vi "ScriptCreateEnumTypedef.vi"(9 "I/O names":string[](array[string]), 11 "Path to Saved File":path) -> ()   [LabVIEW 2014]
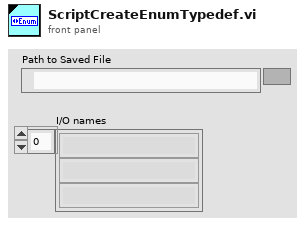
[diagram p1: front panel]
types:
  T1 = enum32{"not a control VI", "control", "typedef", "strict typedef"}
  T2 = enum32{"invalid VI type", "Standard VI", "Control VI", "Global VI", "Polymorphic VI", "Configuration VI", "SubSystem", "Facade VI", "Method VI", "Statechart Diagram VI"}
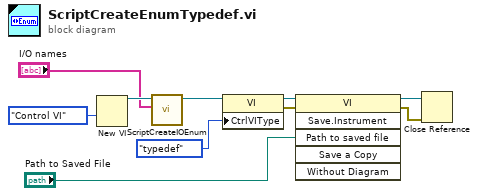
[diagram p0: block diagram]
diagram:
  n1 = New VI(9:T2."Control VI" ("vi type (standard vi)")) -> (3:w10:refnum<vi>)  [unwired: 6 in, 1 out]
  n2 = call "ScriptCreateIOEnum.vi"("I/O names"="I/O names", "VI in"=w10) -> ("VI out"=w8:refnum<vi>)  [unwired: 7 in, 2 out]
  n3 = property class="VI"(reference=w8, "CtrlVIType"=T1."typedef" ("Control VI Type")) -> (reference out=w5:refnum<vi>, error out=w1:errorcluster)  [unwired: 1 in]
  n4 = invoke class="VI" method="Save.Instrument"(reference=w5, error in=w1, "Path to saved file"="Path to Saved File") -> (reference out=w2:refnum<vi>, error out=w3:errorcluster)  [unwired: 3 in, 4 out]
  n5 = Close Reference(reference=w2, error in (no error)=w3) -> ()  [unwired: 1 out]
